vi "HISTOmain.vi"() -> ()   [LabVIEW 2011]
uses:
  MT Scan/SubVIs/hhlib.dll
panel:
  out "Histogram 2":i32[][](graph)
  out "Warnings":string
  out "Resol / ps":dbl format="%.2f"
  in  "Acq.Time /ms":i32=1000 min=1 max=3600000 step=100
  out "Sync Rate":i32
  in  "Syncdiv":enum16{"1", "2", "4", "8"}(ring)
  in  "Binning":i32 min=0 max=10 step=1
  in  "Sync Level":i32=50 min=0 max=800 step=2
  in  "Ch1 Level":i32=50 min=0 max=800 step=10
  in  "Ch1 ZeroX":i32=10 min=0 max=20 step=1
  in  "Sync ZeroX":i32=10 min=0 max=20 step=1
  in  "Sync Offs":i32=-10000 min=-99999 max=99999 step=1
  in  "Ch1 Offs":i32 min=-99999 max=99999 step=1
  in  "Ch2 Level":i32=50 min=0 max=800 step=10
  in  "Ch2 ZeroX":i32=10 min=0 max=20 step=1
  in  "Ch2 Offs":i32 min=-99999 max=99999 step=1
  in  "Ch3 Level":i32=50 min=0 max=800 step=10
  in  "Ch3 ZeroX":i32=10 min=0 max=20 step=1
  in  "Ch3 Offs":i32 min=-99999 max=99999 step=1
  in  "Ch4 Offs":i32 min=-99999 max=99999 step=1
  in  "Ch4 Level":i32=50 min=0 max=800 step=10
  in  "Ch4 ZeroX":i32=10 min=0 max=20 step=1
  out "Serial Num.":string
  out "DeviceIndex":i32=-1
  out "IntegralCount":i32[](array[numeric])
  out "Histogram":u32[][](graph)
  out "Oveflow":bool
  out "DLL Version (must be 1.2)":string caption="DLL Version"
  out "Calibration Status":string
  in  "Run":bool
  in  "done":bool
  out "Initialization Status":string
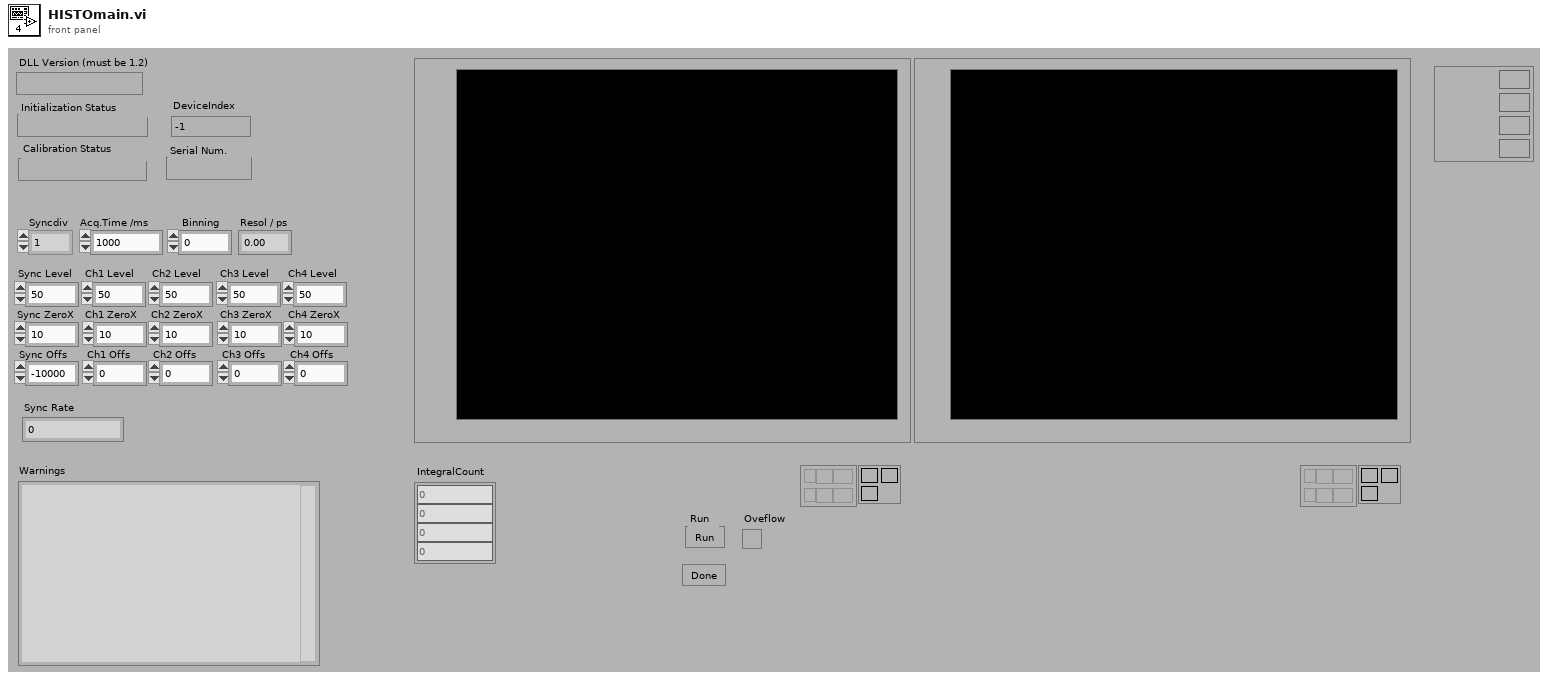
[diagram p1: front panel]
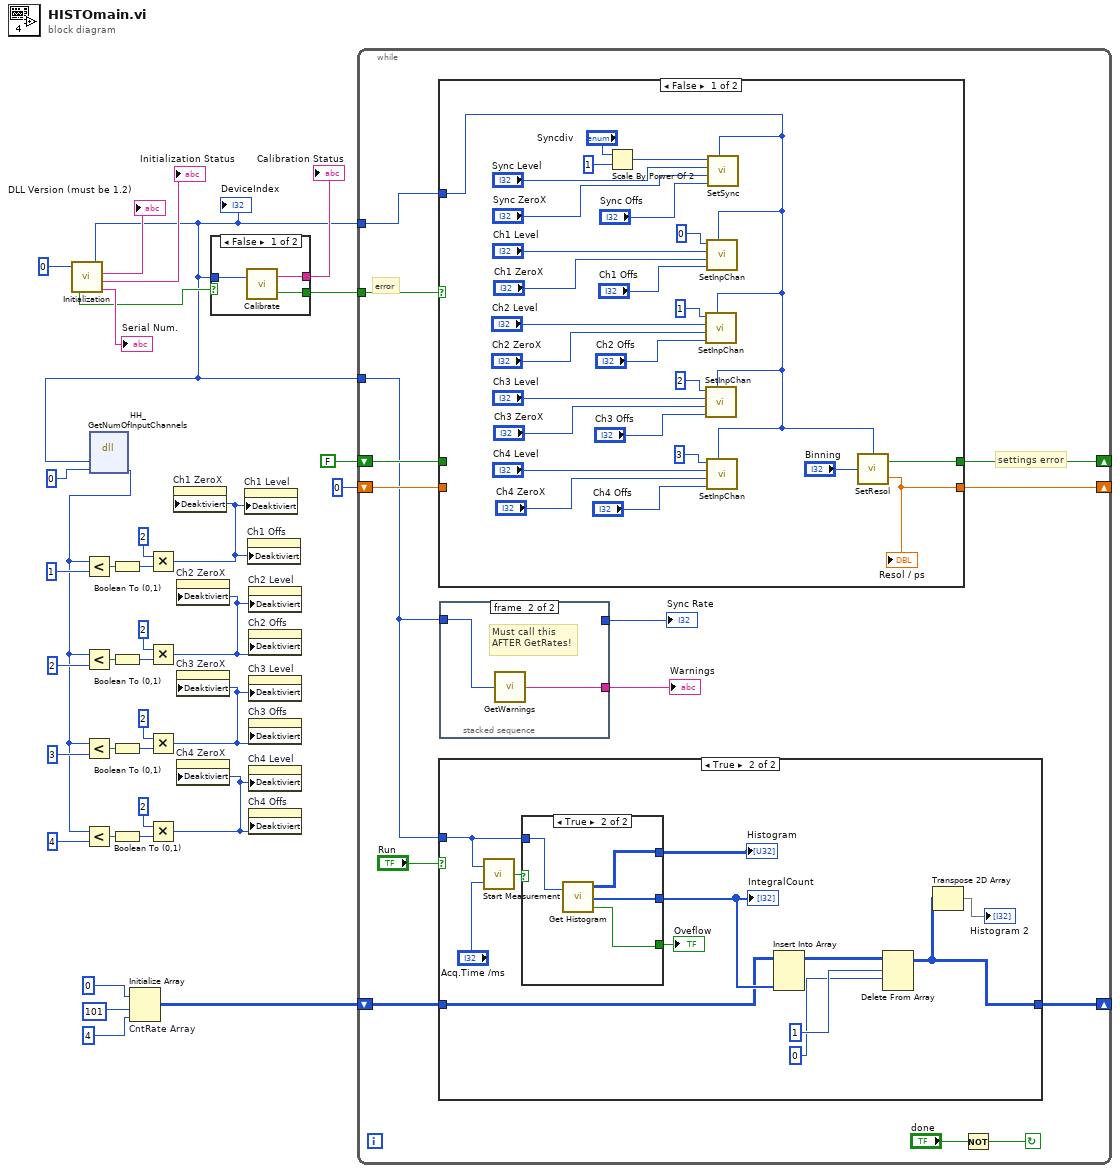
[diagram p0: block diagram]
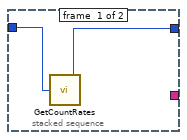
[diagram p2: hidden frame]
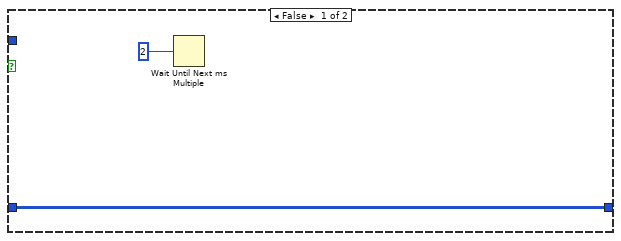
[diagram p3: hidden frame]
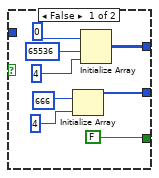
[diagram p4: hidden frame]
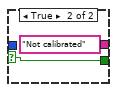
[diagram p6: hidden frame]
diagram:
  # "settings error"
  n1 = call "Initialization.vi"("Mode"=0) -> ("Initialisation Error"=w29:bool, "Deviceindex"=w7:i32, "DLL Version"=→"DLL Version (must be 1.2)":string, "Initialization Status"=→"Initialization Status":string, "Serial[8]"=→"Serial Num.":string)
  "DeviceIndex" <- w7
  n2 = dll-call lib="C:/Users/Core-FCS/Desktop/AbelFCS/MT Scan/SubVIs/hhlib.dll" fn="HH_GetNumOfInputChannels" label="HH_GetNumOfCh"("devidx"=w7, "numch"=0) -> ("numch"=w5:i32)  [unwired: 5 in, 2 out]
  n3 = Less?(x=w5, y=1) -> (x < y?=w26:bool)
  n4 = Less?(x=w5, y=2) -> (x < y?=w21:bool)
  n5 = Less?(x=w5, y=3) -> (x < y?=w17:bool)
  n6 = Less?(x=w5, y=4) -> (x < y?=w13:bool)
  n7 = Boolean To (0,1)(Boolean=w26) -> (0, 1=w25:i16)
  n8 = Boolean To (0,1)(Boolean=w21) -> (0, 1=w22:i16)
  n9 = Boolean To (0,1)(Boolean=w17) -> (0, 1=w18:i16)
  n10 = Boolean To (0,1)(Boolean=w13) -> (0, 1=w14:i16)
  n11 = Initialize Array "CntRate Array"(0, 101, 4) -> (w1:i32[][])
  n12 = Multiply(x=2, y=w25) -> (x*y=w8:i32)
  n13 = Multiply(x=2, y=w22) -> (x*y=w9:i32)
  n14 = Multiply(x=2, y=w18) -> (x*y=w10:i32)
  n15 = Multiply(x=2, y=w14) -> (x*y=w11:i32)
  n16 = property on="Ch1 ZeroX" class="DigNum (strict)"("Deaktiviert"=w8) -> ()  [unwired: 2 in, 2 out]
  n17 = property on="Ch2 ZeroX" class="DigNum (strict)"("Deaktiviert"=w9) -> ()  [unwired: 2 in, 2 out]
  n18 = property on="Ch3 ZeroX" class="DigNum (strict)"("Deaktiviert"=w10) -> ()  [unwired: 2 in, 2 out]
  n19 = property on="Ch4 ZeroX" class="DigNum (strict)"("Deaktiviert"=w11) -> ()  [unwired: 2 in, 2 out]
  n20 = case shown="False" w29 {
    selector: w29 -> [_ w40]
    tunnel: [w39 "Not calibrated"] -> w36
    tunnel: [w38 w40] -> w34
    tunnel: w7 -> [w37 _]
    frame False {
      n21 = call "Calibrate.vi"("Deviceindex"=w37) -> ("Calib Error"=w38:bool, "Status"=w39:string)  [unwired: 1 in]
    }
    frame True {
    }
  }
  "Calibration Status" <- w36
  n22 = property on="Ch1 Level" class="DigNum (strict)"("Deaktiviert"=w8) -> ()  [unwired: 2 in, 2 out]
  n23 = property on="Ch1 Offs" class="DigNum (strict)"("Deaktiviert"=w8) -> ()  [unwired: 2 in, 2 out]
  n24 = property on="Ch2 Level" class="DigNum (strict)"("Deaktiviert"=w9) -> ()  [unwired: 2 in, 2 out]
  n25 = property on="Ch2 Offs" class="DigNum (strict)"("Deaktiviert"=w9) -> ()  [unwired: 2 in, 2 out]
  n26 = property on="Ch3 Level" class="DigNum (strict)"("Deaktiviert"=w10) -> ()  [unwired: 2 in, 2 out]
  n27 = property on="Ch3 Offs" class="DigNum (strict)"("Deaktiviert"=w10) -> ()  [unwired: 2 in, 2 out]
  n28 = property on="Ch4 Level" class="DigNum (strict)"("Deaktiviert"=w11) -> ()  [unwired: 2 in, 2 out]
  n29 = property on="Ch4 Offs" class="DigNum (strict)"("Deaktiviert"=w11) -> ()  [unwired: 2 in, 2 out]
  n30 = while {
    tunnel: w7 -> [w46]
    tunnel: w7 -> [w47]
    tunnel: w34 -> [w51]
    shift-left: 0 -> [w52]
    shift-right: [w53] -> _
    shift-left: FALSE -> [w50]
    shift-right: [w48] -> _
    shift-right: [w43] -> _
    shift-left: w1 -> [w42]
    stop <- w54 continue-if-true
    # "error"
    n31 = case shown="False" w51 {
      tunnel: [w88 w113] -> w48
      tunnel: w50 -> [_ w113]
      tunnel: [w87 w112] -> w53
      tunnel: w52 -> [_ w112]
      tunnel: w47 -> [w86 _]
      frame False {
        n32 = Scale By Power Of 2(n="Syncdiv", x=1) -> (x*2^n=w109:i32)
        n33 = call "SetInpChan.vi"("Channel"=1, "CFD Level"="Ch2 Level", "CFD ZeroX"="Ch2 ZeroX", "Offset"="Ch2 Offs", "DeviceIndex"=w86) -> ()  [unwired: 1 in, 1 out]
        n34 = call "SetInpChan.vi"("Channel"=2, "CFD Level"="Ch3 Level", "CFD ZeroX"="Ch3 ZeroX", "Offset"="Ch3 Offs", "DeviceIndex"=w86) -> ()  [unwired: 1 in, 1 out]
        n35 = call "SetInpChan.vi"("Channel"=0, "CFD Level"="Ch1 Level", "CFD ZeroX"="Ch1 ZeroX", "Offset"="Ch1 Offs", "DeviceIndex"=w86) -> ()  [unwired: 1 in, 1 out]
        n36 = call "SetInpChan.vi"("Channel"=3, "CFD Level"="Ch4 Level", "CFD ZeroX"="Ch4 ZeroX", "Offset"="Ch4 Offs", "DeviceIndex"=w86) -> ()  [unwired: 1 in, 1 out]
        n37 = call "SetSync.vi"("SyncDiv"=w109, "CFD Level"="Sync Level", "CFD ZeroX"="Sync ZeroX", "Offset"="Sync Offs", "DeviceIndex"=w86) -> ()  [unwired: 1 in, 1 out]
        n38 = call "SetResol.vi"("DeviceIndex"=w86, "Binning"="Binning") -> ("Resolution"=w87:dbl, "Error"=w88:bool)  [unwired: 2 in]
        "Resol / ps" <- w87
      }
      frame True {
      }
    }
    n39 = case shown="True" "Run" {
      tunnel: w46 -> [_ w70]
      tunnel: [w60 w62] -> w43
      tunnel: w42 -> [w60 w63]
      frame False {
        n40 = Wait Until Next ms Multiple(millisecond multiple=2) -> ()  [unwired: 1 out]
      }
      frame True {
        n41 = call "Start Measurement.vi"("Acquisition time"="Acq.Time /ms", "DeviceIndex"=w70) -> ("DataValid"=w73:bool)
        n42 = case shown="True" w73 {
          tunnel: [FALSE w85] -> w72
          tunnel: [w75 w84] -> w71
          tunnel: [w74 w83] -> w65
          tunnel: w70 -> [_ w82]
          frame False {
            n43 = Initialize Array(u32 666, 4) -> (w74:u32[])
            n44 = Initialize Array(u32 0, 65536, 4) -> (w75:u32[][])
          }
          frame True {
            n45 = call "Get Histogram.vi"("DeviceIndex"=w82) -> ("Histograms"=w84:u32[][], "IntegralCount"=w83:i32[], "Overflow"=w85:bool)  [unwired: 1 in]
          }
        }
        "Oveflow" <- w72
        "Histogram" <- w71
        "IntegralCount" <- w65
        n46 = Insert Into Array(array=w63, new element=w65) -> (w68:i32[][])  [unwired: 2 in]
        n47 = Delete From Array(array=w68, length=1, index (row)=0) -> (array with subset deleted=w62:i32[][])  [unwired: 1 in, 1 out]
        n48 = Transpose 2D Array(2D array=w62) -> (transposed array=→"Histogram 2":i32[][])
      }
    }
    n49 = stacked-sequence {
      tunnel: w46 -> [w57 w58]
      tunnel: [w56 _] -> w45
      tunnel: [_ w59] -> w44
      frame #0 {
        n50 = call "GetCountRates.vi"("DeviceIndex"=w57) -> ("SyncRate"=w56:i32)  [unwired: 1 out]
      }
      frame #1 {
        # "Must call this\nAFTER GetRates!"
        n51 = call "GetWarnings.vi"("Deviceindex"=w58) -> ("warningstext"=w59:string)
      }
    }
    "Sync Rate" <- w45
    "Warnings" <- w44
    n52 = Not(x="done") -> (.not. x?=w54:bool)
  }
